vi "Set Value.vi"(8 "error in":errorcluster, 10 "Value":variant, 11 "Check Box in":refnum<class "Check Box.lvclass">) -> (0 "error out":errorcluster, 3 "Check Box out":refnum<class "Check Box.lvclass">)   [LabVIEW 2023, in "SourceGrid.lvlib" / "Check Box.lvclass"]
uses:
  Check Box.lvclass
  D:/git/Sourcegrid-LabVIEW/dll/SourceGrid.dll
  dll/SourceGrid.dll
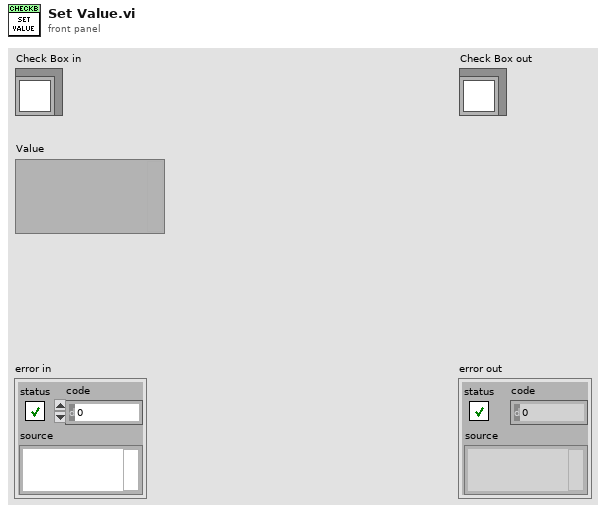
[diagram p1: front panel]
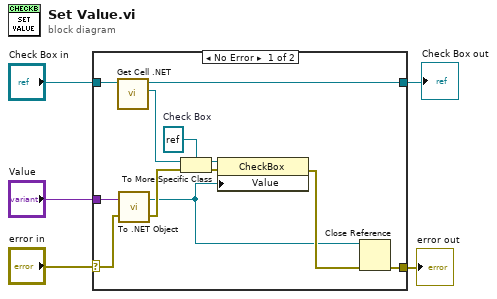
[diagram p0: block diagram]
diagram:
  n1 = case shown="No Error" "error in" {
    selector: "error in" -> [w16 w18]
    tunnel: "Value" -> [w17 _]
    tunnel: "Check Box in" -> [w15 w19]
    tunnel: [w13 w19] -> w2
    tunnel: [w7 w18] -> w1
    frame No Error {
      w11 = refnum<k24> refnum  # Check Box
      n2 = call-dynamic "Get Cell .NET.vi"("Cell in"=w15) -> ("Cell .NET"=w14:refnum<k24>, "Cell out"=w13:refnum<class "Check Box.lvclass">)  [unwired: 9 in]
      n3 = call <vilib>:"To .NET Object.vi"("error in (no error)"=w16, "anything"=w17) -> ("error out"=w10:errorcluster, ".NET object"=w6:refnum<k24>)
      n4 = To More Specific Class(target class=w11, reference=w14, error in=w10) -> (specific class reference=w12:refnum<k24>, error out=w9:errorcluster)
      n5 = property class="CheckBox"(reference=w12, error in=w9, "Value"=w6) -> (error out=w8:errorcluster)  [unwired: 1 out]
      n6 = Close Reference(reference=w6, error in (no error)=w8) -> (error out=w7:errorcluster)
    }
    frame Error {
    }
  }
  "error out" <- w1
  "Check Box out" <- w2
